vi "LB_IndexArray_Tests.vi"(11 "error in":errorcluster) -> (15 "error out":errorcluster)   [LabVIEW 2016, in "DronaTest.lvlib"]
uses:
  DronaTest.lvlib
  APIs/Stimulus/ControlValue/SetValueAuto.vi
  APIs/Stimulus/ControlValue/Controls/Listbox/SetValueByArrayIndex.vi
  APIs/Assert/AssertControlValue/Equal.vi
  APIs/Get/GetControlRef/GetControlRefByPath.vi
  Drona.lvlib
  <vilib>/SLL Toolkit/SLL Debug/SLL Debug.lvlib
  APIs/Stimulus/ControlValue/ControlValue.lvlib
  APIs/Stimulus/ControlValue/Controls/Listbox/StimulusListbox.lvlib
  APIs/Assert/AssertControlValue/AssertControlValue.lvlib
  <vilib>/addons/_JKI Toolkits/Caraya/classes/Assert/Assert.lvclass
  APIs/Get/GetControlRef/GetControlRef.lvlib
  <vilib>/addons/_JKI Toolkits/Caraya/classes/Test/Test.lvclass
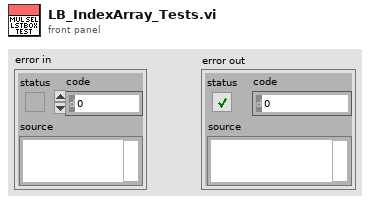
[diagram p1: front panel]
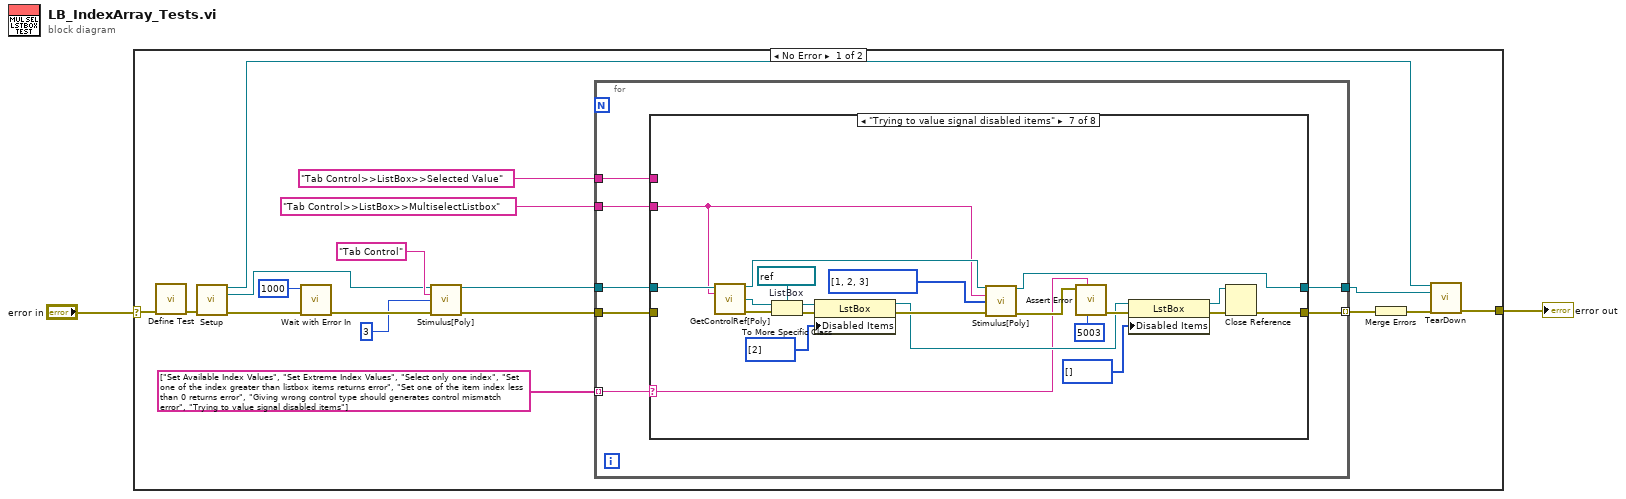
[diagram p0: block diagram]
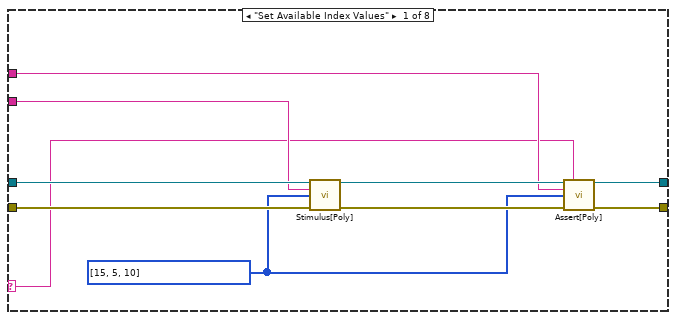
[diagram p2: hidden frame]
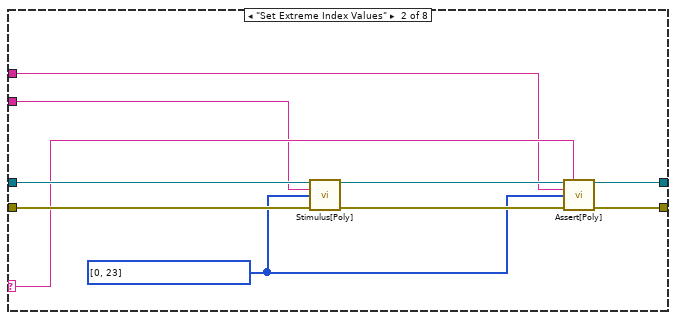
[diagram p3: hidden frame]
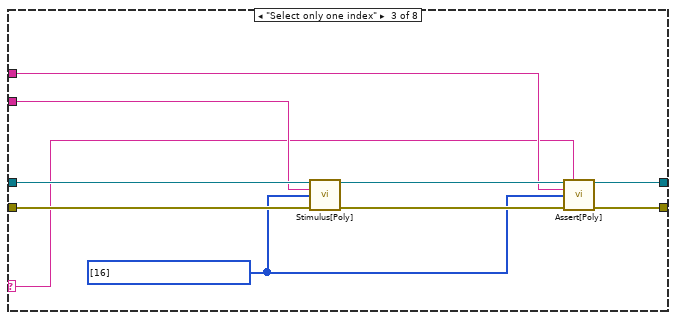
[diagram p4: hidden frame]
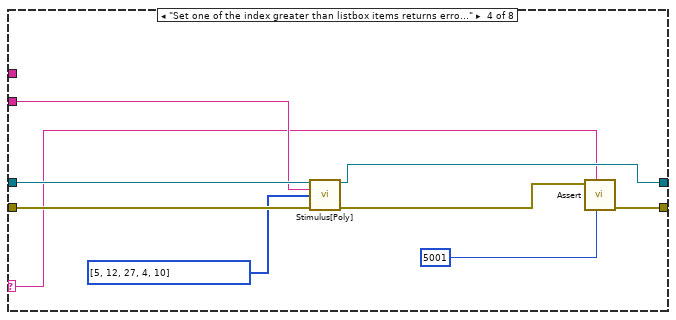
[diagram p5: hidden frame]
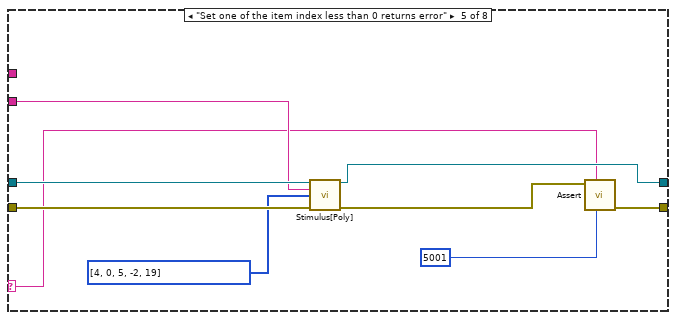
[diagram p6: hidden frame]
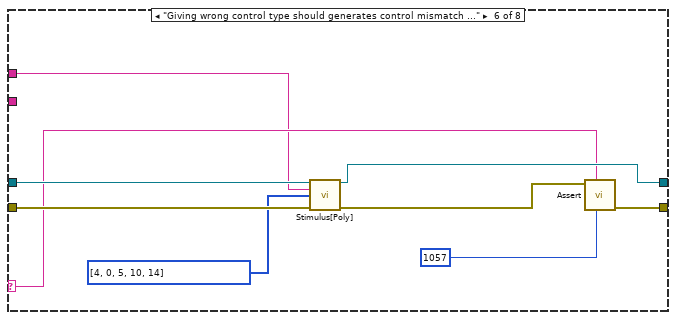
[diagram p7: hidden frame]
diagram:
  n1 = case shown="No Error" "error in" {
    selector: "error in" -> [w3 w108]
    tunnel: [w5 w108] -> w2
    frame No Error {
      n2 = call <vilib>:"Define Test.vi"("error in (no error)"=w3) -> ("error out"=w4:errorcluster)  [unwired: 9 in, 1 out]
      n3 = call "Setup.vi"("error in"=w4) -> ("Application Ref"=w6:refnum<vi>, "VI out"=w10:refnum<vi>, "error out"=w9:errorcluster)  [unwired: 12 in]
      n4 = call <vilib>:"Wait with Error In.vi"("error in (no error)"=w9, "milliseconds to wait"=u32 1000) -> ("error out"=w19:errorcluster)  [unwired: 9 in]
      n5 = call-poly "Stimulus[Poly].vi"("VI Reference In"=w10, "Control Path"="Tab Control", "Value (Signaling)"=3, "error in"=w19) -> ("VI Reference Out"=w15:refnum<vi>, "error out"=w18:errorcluster)  [unwired: 10 in]
      n6 = for {
        tunnel: w18 -> [w27]
        tunnel: w15 -> [w26]
        tunnel: "Tab Control>>ListBox>>MultiselectListbox" ("Control Path") -> [w25]
        tunnel: "Tab Control>>ListBox>>Selected Value" ("Control Path") -> [w24]
        tunnel: [w23] -> w12 mode=indexing
        tunnel: [w22] -> w7
        tunnel: string[] ["Set Available Index Values", "Set Extreme Index Values", "Select only one index", "Set one of the index greater than listbox items returns error", "Set one of the item index less than 0 returns error", "Giving wrong control type should generates control mismatch error", "Trying to value signal disabled items"] -> [w21] mode=indexing
        n7 = case shown="\"Trying to value signal disabled items\"" w21 {
          selector: w21 -> [w28 w40 w48 w60 w69 w79 w90 _]
          tunnel: w27 -> [w37 w47 w57 w66 w75 w84 _ w107]
          tunnel: w26 -> [w36 w46 w56 w65 w74 w83 w87 w106]
          tunnel: w25 -> [w35 w38 w55 w64 w73 _ w85 _]
          tunnel: w24 -> [w32 w39 w52 _ _ w76 _ _]
          tunnel: [w30 w42 w50 w62 w71 w81 w89 w107] -> w23
          tunnel: [w29 w41 w49 w61 w70 w80 w88 w106] -> w22
          frame "Set Available Index Values" {
            w31 = i32[] [15, 5, 10] ("Index Array")
            n8 = call-poly "Stimulus[Poly].vi"("VI Reference In"=w36, "Control Path"=w35, "Index Array"=w31, "Error In"=w37) -> ("VI Reference Out"=w33:refnum<vi>, "Error Out"=w34:errorcluster)  [unwired: 10 in]
            n9 = call-poly "Assert[Poly].vi"("VI Reference In"=w33, "Test Label"=w28, "Control Path"=w32, "Control Value"=w31, "Error In"=w34) -> ("VI Reference Out"=w29:refnum<vi>, "Error Out"=w30:errorcluster)  [unwired: 8 in, 1 out]
          }
          frame "Set Extreme Index Values" {
            w43 = i32[] [0, 23] ("Index Array")
            n10 = call-poly "Stimulus[Poly].vi"("VI Reference In"=w46, "Control Path"=w38, "Index Array"=w43, "Error In"=w47) -> ("VI Reference Out"=w44:refnum<vi>, "Error Out"=w45:errorcluster)  [unwired: 10 in]
            n11 = call-poly "Assert[Poly].vi"("VI Reference In"=w44, "Test Label"=w40, "Control Path"=w39, "Control Value"=w43, "Error In"=w45) -> ("VI Reference Out"=w41:refnum<vi>, "Error Out"=w42:errorcluster)  [unwired: 8 in, 1 out]
          }
          frame "Select only one index" {
            w51 = i32[] [16] ("Index Array")
            n12 = call-poly "Stimulus[Poly].vi"("VI Reference In"=w56, "Control Path"=w55, "Index Array"=w51, "Error In"=w57) -> ("VI Reference Out"=w53:refnum<vi>, "Error Out"=w54:errorcluster)  [unwired: 10 in]
            n13 = call-poly "Assert[Poly].vi"("VI Reference In"=w53, "Test Label"=w48, "Control Path"=w52, "Control Value"=w51, "Error In"=w54) -> ("VI Reference Out"=w49:refnum<vi>, "Error Out"=w50:errorcluster)  [unwired: 8 in, 1 out]
          }
          frame "Set one of the index greater than listbox items returns error" {
            n14 = call-poly "Stimulus[Poly].vi"("VI Reference In"=w65, "Control Path"=w64, "Index Array"=i32[] [5, 12, 27, 4, 10], "Error In"=w66) -> ("VI Reference Out"=w61:refnum<vi>, "Error Out"=w59:errorcluster)  [unwired: 10 in]
            n15 = call-poly <vilib>:"Assert.vi"("error code (1)"=5001, "Label"=w60, "Error?"=w59) -> ("error out"=w62:errorcluster)  [unwired: 7 in, 1 out]
          }
          frame "Set one of the item index less than 0 returns error" {
            n16 = call-poly "Stimulus[Poly].vi"("VI Reference In"=w74, "Control Path"=w73, "Index Array"=i32[] [4, 0, 5, -2, 19], "Error In"=w75) -> ("VI Reference Out"=w70:refnum<vi>, "Error Out"=w68:errorcluster)  [unwired: 10 in]
            n17 = call-poly <vilib>:"Assert.vi"("error code (1)"=5001, "Label"=w69, "Error?"=w68) -> ("error out"=w71:errorcluster)  [unwired: 7 in, 1 out]
          }
          frame "Giving wrong control type should generates control mismatch error" {
            n18 = call-poly "Stimulus[Poly].vi"("VI Reference In"=w83, "Control Path"=w76, "Index Array"=i32[] [4, 0, 5, 10, 14], "Error In"=w84) -> ("VI Reference Out"=w80:refnum<vi>, "Error Out"=w78:errorcluster)  [unwired: 10 in]
            n19 = call-poly <vilib>:"Assert.vi"("error code (1)"=1057, "Label"=w79, "Error?"=w78) -> ("error out"=w81:errorcluster)  [unwired: 7 in, 1 out]
          }
          frame "Trying to value signal disabled items" {
            w104 = refnum<vi> refnum  # ListBox
            n20 = call-poly "GetControlRef[Poly].vi"("VI Reference In"=w87, "Control Path"=w85) -> ("VI Reference Out"=w99:refnum<vi>, "Ctl Refnum"=w98:refnum<vi>, "error out"=w100:errorcluster)  [unwired: 11 in]
            n21 = To More Specific Class(target class=w104, reference=w98, error in=w100) -> (specific class reference=w103:refnum<vi>, error out=w105:errorcluster)
            n22 = property class="LstBox"(reference=w103, error in=w105, "Disabled Items"=i32[] [2]) -> (reference out=w92:refnum<vi>, error out=w101:errorcluster)
            n23 = call-poly "Stimulus[Poly].vi"("VI Reference In"=w99, "Control Path"=w85, "Index Array"=i32[] [1, 2, 3], "Error In"=w101) -> ("VI Reference Out"=w88:refnum<vi>, "Error Out"=w96:errorcluster)  [unwired: 10 in]
            n24 = call <vilib>:"Assert Error.vi"("error code (1)"=5003, "Label"=w90, "Error?"=w96) -> ("error out"=w95:errorcluster)  [unwired: 7 in, 1 out]
            n25 = property class="LstBox"(reference=w92, error in=w95, "Disabled Items"=i32[] []) -> (reference out=w93:refnum<vi>, error out=w94:errorcluster)
            n26 = Close Reference(reference=w93, error in (no error)=w94) -> (error out=w89:errorcluster)
          }
          frame Default {
          }
        }
      }
      n27 = Merge Errors(w12) -> (w8:errorcluster)
      n28 = call "TearDown.vi"("Application Ref"=w6, "VI in"=w7, "error in (no error)"=w8) -> ("error out"=w5:errorcluster)  [unwired: 12 in]
    }
    frame Error {
    }
  }
  "error out" <- w2
